vi "iRobot Initialize.vi"(11 "UART port in":T1) -> (0 "error out":errorcluster, 3 "UART port out":T1)   [LabVIEW 2010]
doc: "Open UART serial port and initilize iRobot.\n\nThis VI both writes to AND reads from the serial port."
uses:
  UART/UART Port Type.ctl
  Actuator/Actuator Controls/iRobot LED.ctl
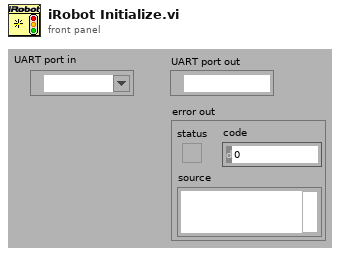
[diagram p1: front panel]
types:
  T1 = typedef "UART Port Type.ctl" = refnum<visa-resource-name>
  T2 = typedef "iRobot LED.ctl" = u8
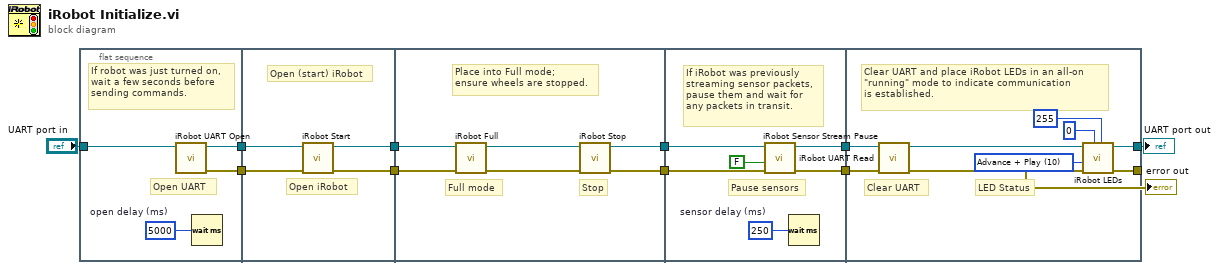
[diagram p0: block diagram]
diagram:
  n1 = flat-sequence {
    tunnel: [w15] -> w4
    tunnel: "UART port in" -> [w14]
    tunnel: [w12] -> w2
    tunnel: w4 -> [w19]
    tunnel: [w18] -> w3
    tunnel: w2 -> [w17]
    tunnel: [w16] -> w1
    tunnel: [w24] -> w9
    tunnel: w3 -> [w21]
    tunnel: w1 -> [w20]
    tunnel: [w22] -> w7
    tunnel: [w30] -> w11
    tunnel: w9 -> [w31]
    tunnel: w7 -> [w27]
    tunnel: [w26] -> w6
    tunnel: [w37] -> w10
    tunnel: w11 -> [w38]
    tunnel: w6 -> [w36]
    tunnel: [w32] -> w5
    frame #0 {
      w13 = u32 5000  # open delay (ms)
      # "If robot was just turned on,\nwait a few seconds before\nsending commands."
      # "Open UART"
      n2 = call "iRobot UART Open.vi"("UART port in"=w14) -> ("error out"=w12:errorcluster, "UART port out"=w15:T1)  [unwired: 9 out]
      n3 = Wait (ms)(milliseconds to wait=w13) -> ()  [unwired: 1 out]
    }
    frame #1 {
      # "Open (start) iRobot"
      # "Open iRobot"
      n4 = call "iRobot Start.vi"("error in"=w17, "UART port in"=w19) -> ("error out"=w16:errorcluster, "UART port out"=w18:T1)  [unwired: 8 out]
    }
    frame #2 {
      # "Place into Full mode;\nensure wheels are stopped."
      # "Full mode"
      # "Stop"
      n5 = call "iRobot Full.vi"("error in"=w20, "UART port in"=w21) -> ("error out"=w23:errorcluster, "UART port out"=w25:T1)  [unwired: 8 out]
      n6 = call "iRobot Stop.vi"("error in"=w23, "UART port in"=w25) -> ("error out"=w22:errorcluster, "UART port out"=w24:T1)  [unwired: 8 out]
    }
    frame #3 {
      w29 = u32 250  # sensor delay (ms)
      # "If iRobot was previously\nstreaming sensor packets,\npause them and wait for\nany packets in transit."
      # "Pause sensors"
      n7 = call "iRobot Sensor Stream Pause.vi"("error in"=w27, "Resume?"=FALSE, "UART port in"=w31) -> ("error out"=w26:errorcluster, "UART port out"=w30:T1)  [unwired: 1 in, 6 out]
      n8 = Wait (ms)(milliseconds to wait=w29) -> ()  [unwired: 1 out]
    }
    frame #4 {
      w39 = T2 10 items=["None"=0, "Advance"=8, "Play"=2, "Advance + Play"=10] ("LEDs on")
      # "Clear UART and place iRobot LEDs in an all-on\n\"running\" mode to indicate communication\nis established."
      # "Clear UART"
      # "LED Status"
      n9 = call "iRobot UART Read.vi"("error in"=w36, "UART port in"=w38) -> ("error out"=w35:errorcluster, "UART port out"=w40:T1)  [unwired: 8 out]
      n10 = call "iRobot LEDs.vi"("Power LED Intensity (0-255)"=u8 255 ("Power LED Color (R-G)"), "Power LED Color (G[0]-R[255])"=u8 0, "error in"=w35, "LEDs on"=w39, "UART port in"=w40) -> ("error out"=w32:errorcluster, "UART port out"=w37:T1)  [unwired: 3 in, 2 out]
    }
  }
  "UART port out" <- w10
  "error out" <- w5
